vi "Create Messages.vi"(7 "App":refnum<vi>, 8 "error in (no error)":errorcluster, 11 "LV-Protoc in":refnum<class "LV-Protoc.lvclass">) -> (0 "error out":errorcluster, 3 "LV-Protoc out":refnum<class "LV-Protoc.lvclass">)   [LabVIEW 2020, in "LV-Protoc.lvlib" / "LV-Protoc.lvclass"]
uses:
  LV-Protoc.lvclass
  LV-Proto/Message.ctl
  LV-Proto/Field.ctl
  LV-Proto/Type.ctl
  LV-Proto/Proto Type.ctl
  LV-Protoc.lvclass/LV-Protoc.ctl
  LV-Proto/LV-Proto.lvlib
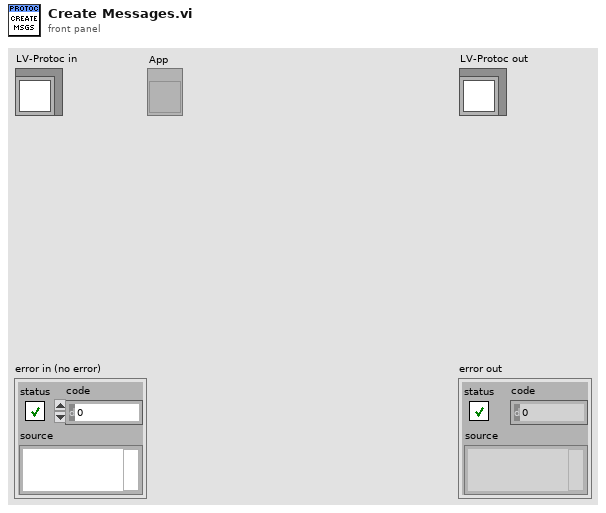
[diagram p1: front panel]
types:
  T1 = typedef "LV-Proto.lvlib/Message.ctl" = cluster{"Name":string, "Fields":T2[], "Reserved Numbers":u32[], "Reserved Names":string[]}
  T2 = typedef "LV-Proto.lvlib/Field.ctl" = cluster{"Name":string, "Number":u32, "Optional":bool, "Repeated":bool, "Type":T3, "Key Type":T3, "Value Type":T3}
  T3 = typedef "LV-Proto.lvlib/Type.ctl" = cluster{"Type":T4, "Subtype":string}
  T4 = typedef "LV-Proto.lvlib/Proto Type.ctl" = enum16{"UNKNOWN", "double", "float", "int32", "int64", "uint32", "uint64", "sint32", "sint64", "fixed32", "fixed64", "sfixed32", "sfixed64", "bool", "string", "bytes", "enum", "map", "message"}
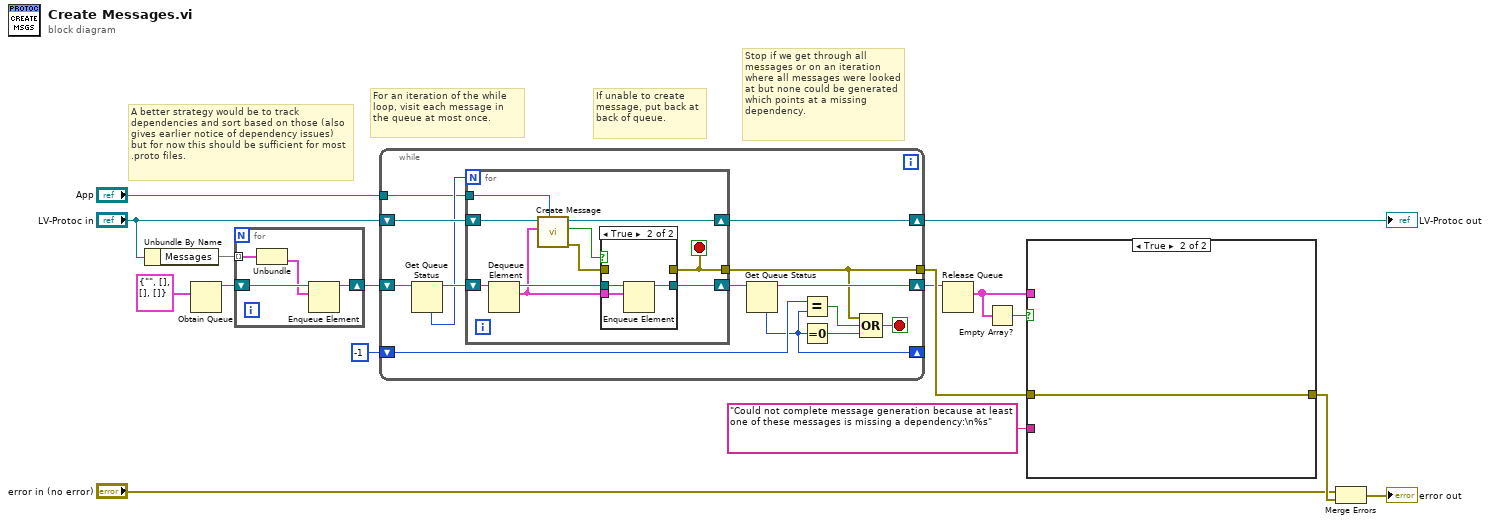
[diagram p0: block diagram]
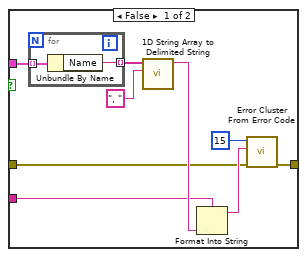
[diagram p3: hidden frame]
diagram:
  # "If unable to create message, put back at back of queue."
  # "Stop if we get through all messages or on an iteration where all messages were looked at but none could be generated which points at a missing dependency."
  # "For an iteration of the while loop, visit each message in the queue at most once."
  # "A better strategy would be to track dependencies and sort based on those (also gives earlier notice of dependency issues) but for now this should be sufficient for most .proto files."
  n1 = Unbundle By Name("LV-Protoc in") -> ("Messages"=w13:map{string, T1})
  n2 = Obtain Queue(element data type=T1 {"Name"="", "Fields"=[], "Reserved Numbers"=[], "Reserved Names"=[]} ("Message")) -> (queue out=w14:refnum<queue>)  [unwired: 4 in, 2 out]
  n3 = for {
    shift-right: [w17] -> w12
    shift-left: w14 -> [w19]
    tunnel: w13 -> [w20] mode=indexing
    n4 = Unbundle(w20) -> ("Message"=w18:T1)  [unwired: 1 out]
    n5 = Enqueue Element(queue=w19, element=w18) -> (queue out=w17:refnum<queue>)  [unwired: 2 in, 2 out]
  }
  n6 = while {
    shift-right: [w34] -> w9
    shift-left: w12 -> [w33]
    shift-right: [w24] -> w10
    shift-left: "LV-Protoc in" -> [w26]
    shift-right: [w30] -> _
    shift-left: -1 -> [w32]
    tunnel: [w22] -> w16
    tunnel: "App" -> [w21]
    stop <- w29 stop-if-true
    n7 = Get Queue Status(queue=w33) -> (queue out=w27:refnum<queue>, # elements in queue=w25:i32)  [unwired: 2 in, 6 out]
    n8 = for {
      N: w25 -> [_]
      shift-right: [w43] -> w28
      shift-left: w27 -> [w42]
      shift-right: [w39] -> w24
      shift-left: w26 -> [w41]
      tunnel: [w36] -> w22
      tunnel: w21 -> [w35]
      stop <- w36 stop-if-true
      n9 = Dequeue Element(queue=w42) -> (queue out=w44:refnum<queue>, element=w40:T1)  [unwired: 2 in, 2 out]
      n10 = call "Create Message.vi"("App"=w35, "Message"=w40, "LV-Protoc in"=w41) -> ("error out"=w37:errorcluster, "Missing Deps"=w38:bool, "LV-Protoc out"=w39:refnum<class "LV-Protoc.lvclass">)  [unwired: 6 in]
      n11 = case shown="True" w38 {
        tunnel: w40 -> [_ w48]
        tunnel: w44 -> [w46 w49]
        tunnel: [w46 w47] -> w43
        tunnel: w37 -> [w45 _]
        tunnel: [w45 _] -> w36
        frame False {
        }
        frame True {
          n12 = Enqueue Element(queue=w49, element=w48) -> (queue out=w47:refnum<queue>)  [unwired: 2 in, 2 out]
        }
      }
    }
    n13 = Get Queue Status(queue=w28) -> (queue out=w34:refnum<queue>, # elements in queue=w30:i32)  [unwired: 2 in, 6 out]
    n14 = Equal?(x=w32, y=w30) -> (x = y?=w23:bool)
    n15 = Equal To 0?(x=w30) -> (x = 0?=w31:bool)
    n16 = Compound Arithmetic op=OR(w22, w23, w31) -> (w29:bool)
  }
  "LV-Protoc out" <- w10
  n17 = Release Queue(queue=w9) -> (remaining elements=w6:T1[])  [unwired: 2 in, 2 out]
  n18 = Empty Array?(array=w6) -> (empty?=w7:bool)
  n19 = case shown="True" w7 {
    tunnel: w6 -> [w58 _]
    tunnel: [w52 w61] -> w5
    tunnel: w16 -> [w51 w61]
    tunnel: "Could not complete message generation because at least one of these messages is missing a dependency:\n%s" -> [w50 _]
    frame False {
      n20 = for {
        tunnel: w58 -> [w60] mode=indexing
        tunnel: [w59] -> w57 mode=indexing
        n21 = Unbundle By Name(w60) -> ("Name"=w59:string)
      }
      n22 = call <vilib>:"1D String Array to Delimited String.vi"("delimiter"=", ", "string array"=w57) -> ("delimited string"=w54:string)  [unwired: 9 in]
      n23 = Format Into String(format string=w50, w54) -> (resulting string=w53:string)  [unwired: 2 in, 1 out]
      n24 = call <vilib>:"Error Cluster From Error Code.vi"("error in (no error)"=w51, "error message (\"\")"=w53, "error code (0)"=15) -> ("error out"=w52:errorcluster)  [unwired: 6 in]
    }
    frame True {
    }
  }
  n25 = Merge Errors("error in (no error)", w5) -> (→"error out":errorcluster)
